vi "Disable Structure.vi"() -> ()   [LabVIEW 2020]
panel:
  out "Output":dbl
  in  "Numeric 2":dbl
  in  "Numeric":dbl
  # "Disable Structure"
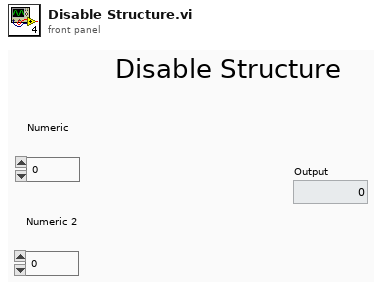
[diagram p1: front panel]
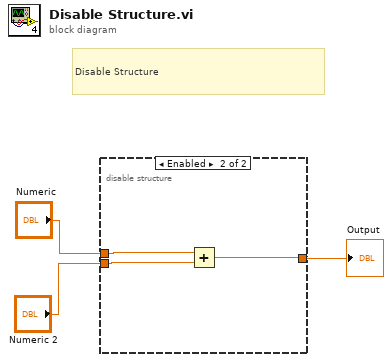
[diagram p0: block diagram]
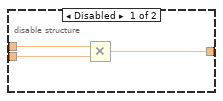
[diagram p2: hidden frame]
diagram:
  # "Disable Structure"
  n1 = disable-structure shown="Enabled" {
    disable-tunnel: "Numeric" -> [w6 w9]
    disable-tunnel: "Numeric 2" -> [w5 w8]
    disable-tunnel: [w4 w7] -> w1
    frame Disabled {
      n2 = Multiply(x=w6, y=w5) -> (x*y=w4:dbl)
    }
    frame Enabled {
      n3 = Add(x=w9, y=w8) -> (x+y=w7:dbl)
    }
  }
  "Output" <- w1
